vi "Estructuras Labview 1.vi"() -> ()   [LabVIEW 2022 SP3]
panel:
  out "Operacion":string
  out "Resta":bool
  out "Suma":bool
  out "Resultado":dbl
  in  "Numeric 2":dbl
  in  "Numeric 1":dbl
  in  "Boolean":bool
  out "Iteraciones":i32
  in  "Stop Button":bool
  # "Se pide diseñar una claculadora de 2 operaciones"
  # "True : Resta\nFalse : Suma"
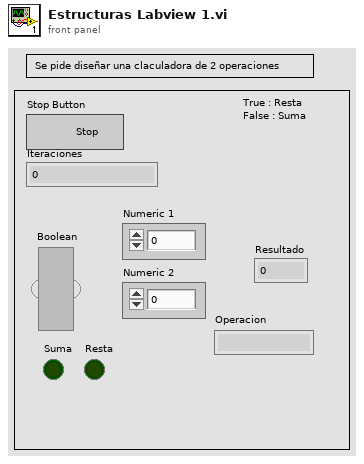
[diagram p1: front panel]
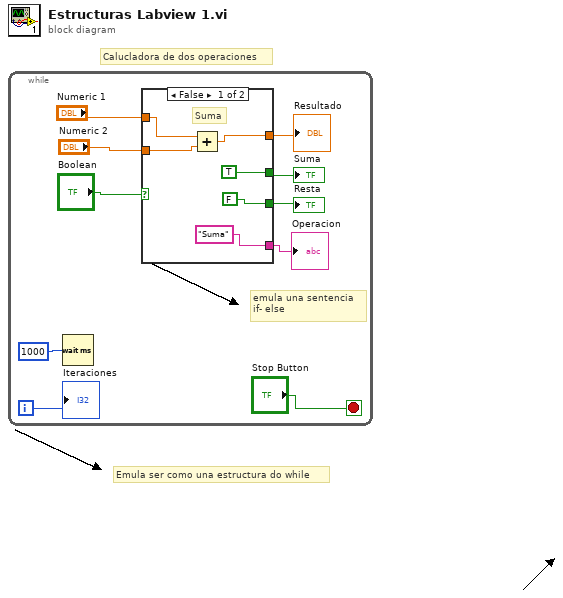
[diagram p0: block diagram]
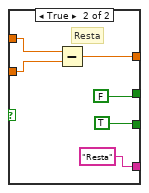
[diagram p2: hidden frame]
diagram:
  # "Emula ser como una estructura do while"
  # "Calucladora de dos operaciones"
  n1 = while {
    i -> [w9]
    stop <- "Stop Button" stop-if-true
    # "emula una sentencia \nif- else"
    n2 = Wait (ms)(milliseconds to wait=u32 1000) -> ()  [unwired: 1 out]
    n3 = case shown="False" "Boolean" {
      tunnel: "Numeric 1" -> [w15 w22]
      tunnel: "Numeric 2" -> [w14 w21]
      tunnel: [w16 w20] -> w5
      tunnel: [TRUE FALSE] -> w4
      tunnel: [FALSE TRUE] -> w3
      tunnel: ["Suma" "Resta"] -> w2
      frame False {
        # "Suma"
        n4 = Add(x=w15, y=w14) -> (x+y=w16:dbl)
      }
      frame True {
        # "Resta"
        n5 = Subtract(x=w22, y=w21) -> (x-y=w20:dbl)
      }
    }
    "Resultado" <- w5
    "Suma" <- w4
    "Resta" <- w3
    "Operacion" <- w2
    "Iteraciones" <- w9
  }
